vi "ExampleInstrument.TestLauncher.vi"() -> ()   [LabVIEW 2016, in "ExampleInstrument.lvclass"]
uses:
  ExampleInstrument.lvclass
  <vilib>/JKI/JKI SMO/SMO/Typedefs/SMOState --Enum.ctl
  C:/user/patrick/hg/levylab_inst/lvsrc/SMOs/Instrument/Instrument.lvclass
  C:/Program Files (x86)/National Instruments/LabVIEW 2016/vi.lib/JKI/JKI SMO/SMO/SMO.lvclass
  Example Instrument UI/ExampleInstrument.UI.lvclass
  C:/Program Files (x86)/National Instruments/LabVIEW 2016/vi.lib/JKI/JKI SMO/SMO.UI/SMO.UI.lvclass
  lvsrc/SMOs/Instrument/Instrument.lvclass/Instrument.ctl
  <vilib>/JKI/JKI SMO/SMO/SMO.lvclass
  <vilib>/JKI/JKI SMO/SMO.UI/SMO.UI.lvclass
  lvsrc/SMOs/Instrument/Instrument.lvclass
panel:
  in  "Debug Mode?":bool
  out "UI SMO State":T1
  out "SMO State":T1
  out "error out":errorcluster
  in  "Stop":bool
  # "Example Instrument SMO Test Launcher"
  # "For instructions on how to use the JKI State Machine Objects, examples and video tutorials, visit:\nhttp://jki.net/state-machine-objects/\n\nJKI State Machine Objects™\nhttp://jki.net/state-machine-objects/\nCopyright (C) 2005-2015, JKI <info@jki.net>\nALL RIGHTS RESERVED"
  # "Starting Example Instrument..."
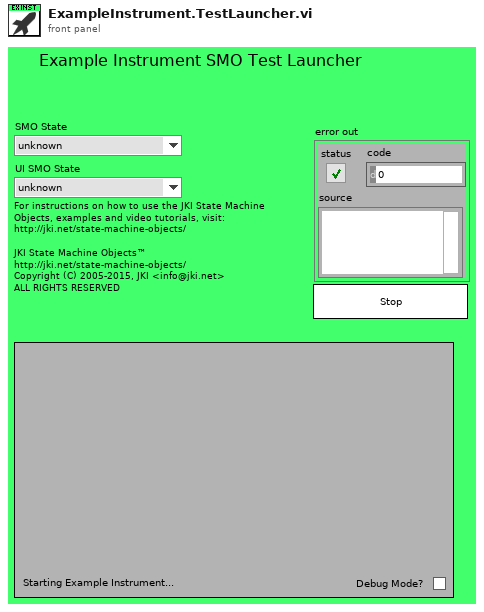
[diagram p1: front panel]
types:
  T1 = typedef "SMO.lvclass/SMOState --Enum.ctl" = enum16{"unknown", "Created", "Started", "Stopped"}
  T2 = typedef "SMO.lvclass/Public Events.ctl" = cluster{"Error":refnum<user-event>, "State":refnum<user-event>, "Reserve State":refnum<user-event>}
  T3 = cluster{"Event Registration Refnum":refnum<event-registration>, "Event Registration Refnum":refnum<event-registration>}
  T4 = enum32{"Invalid", "Standard", "Closed", "Hidden", "Minimized", "Maximized"}
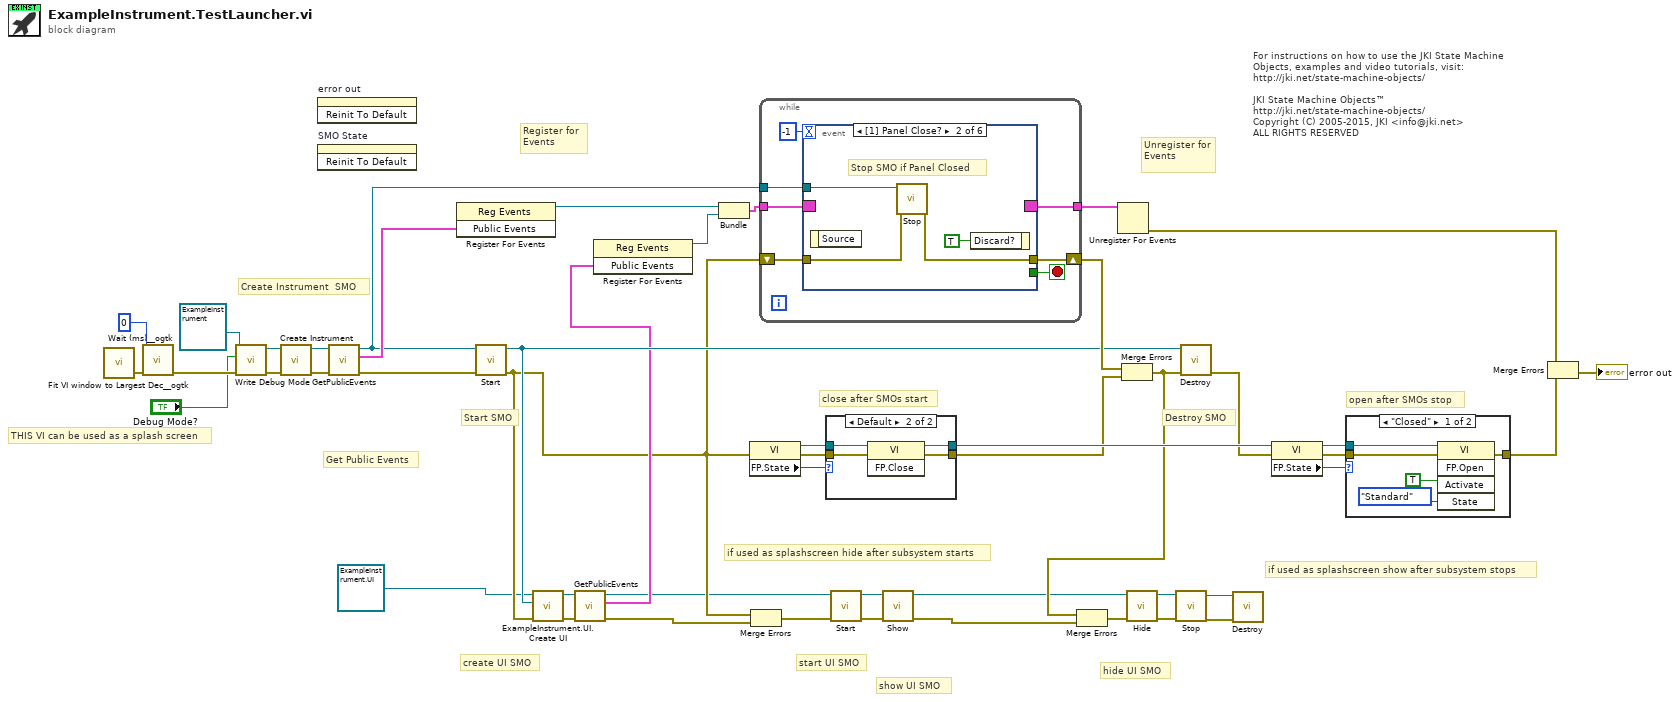
[diagram p0: block diagram]
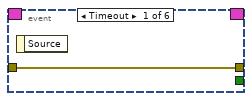
[diagram p4: hidden frame]
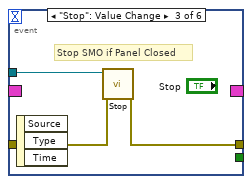
[diagram p5: hidden frame]
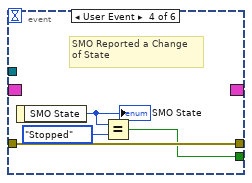
[diagram p6: hidden frame]
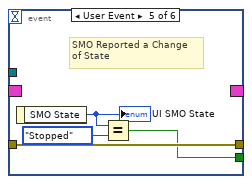
[diagram p7: hidden frame]
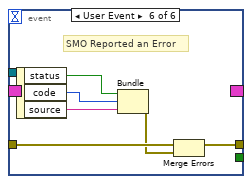
[diagram p8: hidden frame]
diagram:
  # "open after SMOs stop"
  # "close after SMOs start"
  # "hide UI SMO"
  # "show UI SMO"
  # "start UI SMO"
  # "create UI SMO"
  # "if used as splashscreen show after subsystem stops"
  # "if used as splashscreen hide after subsystem starts"
  # "THIS VI can be used as a splash screen"
  # "Get Public Events"
  # "Start SMO"
  # "Destroy SMO"
  # "Create Instrument  SMO"
  # "Unregister for Events"
  # "Register for Events"
  # "For instructions on how to use the JKI State Machine Objects, examples and video tutorials, visit:\nhttp://jki.net/state-machine-objects/\n\nJKI State Machine Objects™\nhttp://jki.net/state-machine-objects/\nCopyright (C) 2005-2015, JKI <info@jki.net>\nALL RIGHTS RESERVED"
  n1 = call <userlib>:"Fit VI window to Largest Dec__ogtk.vi"() -> ("error out"=w35:errorcluster)  [unwired: 6 in, 1 out]
  n2 = call <userlib>:"Wait (ms)__ogtk.vi"("error in (no error)"=w35, "milliseconds to wait"=u32 0) -> ("error out"=w3:errorcluster)  [unwired: 8 in, 1 out]
  n3 = call "Write Debug Mode.vi"("error in (no error)"=w3, "Debug Mode?"="Debug Mode?", "Instrument in"=refnum<class "ExampleInstrument.lvclass"> refnum ("SMO.Template.lvclass")) -> ("error out"=w2:errorcluster, "Instrument out"=w4:refnum<class "ExampleInstrument.lvclass">)  [unwired: 7 in]
  n4 = call-dynamic "Create Instrument.vi"("error in (no error)"=w2, "Instrument in"=w4) -> ("error out"=w42:errorcluster, "Instrument out"=w43:refnum<class "ExampleInstrument.lvclass">)  [unwired: 8 in]
  n5 = invoke on="error out" class="Clust (strict)" method="Reinit To Default"() -> ()  [unwired: 3 in, 3 out]
  n6 = invoke on="SMO State" class="Enum (strict)" method="Reinit To Default"() -> ()  [unwired: 3 in, 3 out]
  n7 = call <vilib>:"GetPublicEvents.vi"("error in (no error)"=w42, "SMO"=w43) -> ("error out"=w41:errorcluster, "Public Events"=w45:T2, "SMO out"=w44:refnum<class "ExampleInstrument.lvclass">)  [unwired: 7 in]
  n8 = register-events(w45) -> (reference out=w34:refnum<event-registration>)  [unwired: 2 in, 1 out]
  n9 = call <vilib>:"Start.vi"("error in (no error)"=w41, "SMO"=w44) -> ("error out"=w27:errorcluster, "SMO out"=w32:refnum<class "ExampleInstrument.lvclass">)  [unwired: 8 in]
  n10 = call "ExampleInstrument.UI.Create UI.vi"("error in (no error)"=w27, "Instrument in"=w32, "Example Instrument UI in"=refnum<class "ExampleInstrument.UI.lvclass"> refnum ("ExampleInstrument.UI.lvclass")) -> ("error out"=w30:errorcluster, "Example Instrument UI out"=w29:refnum<class "ExampleInstrument.UI.lvclass">)  [unwired: 7 in]
  n11 = call <vilib>:"GetPublicEvents.vi"("error in (no error)"=w30, "SMO"=w29) -> ("error out"=w21:errorcluster, "Public Events"=w28:T2, "SMO out"=w22:refnum<class "ExampleInstrument.UI.lvclass">)  [unwired: 7 in]
  n12 = register-events(w28) -> (reference out=w31:refnum<event-registration>)  [unwired: 2 in, 1 out]
  n13 = Bundle("Event Registration Refnum"=w34, "Event Registration Refnum"=w31) -> (w33:T3)  [unwired: 1 in]
  n14 = property class="VI"(error in=w27) -> (reference out=w12:refnum<vi>, error out=w13:errorcluster, "FP.State"=w11:T4)  [unwired: 1 in]
  n15 = Merge Errors(w27, w21) -> (w26:errorcluster)
  n16 = while {
    shift-right: [w54] -> w40
    shift-left: w27 -> [w53]
    tunnel: w33 -> [w52]
    tunnel: [w51] -> w48
    tunnel: w44 -> [w50]
    stop <- w55 stop-if-true
    n17 = event shown="[1] Panel Close?" {
      selector: w52 -> [_ _ _ _ _ _]
      dyn-events: [_ _ _ _ _ _] -> w51
      timeout: -1 -> [_ _ _ _ _ _]
      tunnel: [_ _ _ w64 w68 _] -> w55
      tunnel: w50 -> [_ w60 w63 _ _ _]
      tunnel: [w56 w59 w62 w67 w71 w75] -> w54
      tunnel: w53 -> [w56 w58 w61 w67 w71 w73]
      event Timeout {
        n18 = event-data() -> ()  [unwired: 1 in, 1 out]
      }
      event Panel Close? {
        # "Stop SMO if Panel Closed"
        n19 = event-data() -> ()  [unwired: 1 in, 1 out]
        n20 = call <vilib>:"Stop.vi"("error in (no error)"=w58, "SMO"=w60) -> ("error out"=w59:errorcluster)  [unwired: 8 in, 1 out]
        n21 = event-data("Discard?"=TRUE ("OK")) -> ()  [unwired: 1 in, 1 out]
      }
      event "Stop": Value Change {
        # "Stop SMO if Panel Closed"
        n22 = event-data() -> ()  [unwired: 1 in, 3 out]
        n23 = call <vilib>:"Stop.vi"("error in (no error)"=w61, "SMO"=w63) -> ("error out"=w62:errorcluster)  [unwired: 8 in, 1 out]
      }
      event User Event {
        # "SMO Reported a Change\nof State"
        n24 = event-data() -> ("SMO State"=w66:T1)  [unwired: 1 in]
        "SMO State" <- w66
        n25 = Equal?(x=w66, y=SMOState_--Enum."Stopped") -> (x = y?=w64:bool)
      }
      event User Event {
        # "SMO Reported a Change\nof State"
        n26 = event-data() -> ("SMO State"=w70:T1)  [unwired: 1 in]
        "UI SMO State" <- w70
        n27 = Equal?(x=w70, y=SMOState_--Enum."Stopped") -> (x = y?=w68:bool)
      }
      event User Event {
        # "SMO Reported an Error"
        n28 = event-data() -> ("status"=w74:bool, "code"=w77:i32, "source"=w76:string)  [unwired: 1 in]
        n29 = Bundle("status"=w74, "code"=w77, "source"=w76) -> (w72:errorcluster)  [unwired: 1 in]
        n30 = Merge Errors(w73, w72) -> (w75:errorcluster)
      }
    }
  }
  n31 = case shown="Default" w11 {
    tunnel: [w79 w83] -> w36
    tunnel: w13 -> [w79 w82]
    tunnel: w12 -> [w78 w81]
    tunnel: [w78 w80] -> w39
    frame "Invalid", "Closed" {
    }
    frame Default {
      n32 = invoke class="VI" method="FP.Close"(reference=w81, error in=w82) -> (reference out=w80:refnum<vi>, error out=w83:errorcluster)  [unwired: 1 in, 1 out]
    }
  }
  n33 = call <vilib>:"Start.vi"("error in (no error)"=w26, "SMO"=w22) -> ("error out"=w20:errorcluster, "SMO out"=w19:refnum<class "ExampleInstrument.UI.lvclass">)  [unwired: 8 in]
  n34 = call <vilib>:"Show.vi"("error in (no error)"=w20, "SMO.UI"=w19) -> ("error out"=w18:errorcluster, "SMO.UI out"=w14:refnum<class "ExampleInstrument.UI.lvclass">)  [unwired: 8 in]
  n35 = Unregister For Events(event registration refnum=w48) -> (error out=w47:errorcluster)  [unwired: 1 in]
  n36 = Merge Errors(w40, w36) -> (w23:errorcluster)
  n37 = Merge Errors(w23, w18) -> (w15:errorcluster)
  n38 = call <vilib>:"Hide.vi"("error in (no error)"=w15, "SMO.UI"=w14) -> ("error out"=w17:errorcluster, "SMO.UI out"=w16:refnum<class "ExampleInstrument.UI.lvclass">)  [unwired: 8 in]
  n39 = call <vilib>:"Stop.vi"("error in (no error)"=w17, "SMO"=w16) -> ("error out"=w25:errorcluster, "SMO out"=w24:refnum<class "ExampleInstrument.UI.lvclass">)  [unwired: 8 in]
  n40 = call <vilib>:"Destroy.vi"("error in (no error)"=w23, "SMO"=w32) -> ("error out"=w38:errorcluster)  [unwired: 9 in]
  n41 = call <vilib>:"Destroy.vi"("error in (no error)"=w25, "SMO"=w24) -> ()  [unwired: 9 in, 1 out]
  n42 = property class="VI"(reference=w39, error in=w38) -> (reference out=w9:refnum<vi>, error out=w10:errorcluster, "FP.State"=w8:T4)
  n43 = case shown="\"Closed\"" w8 {
    tunnel: [w86 w89] -> w37
    tunnel: w10 -> [w85 w89]
    tunnel: w9 -> [w84 _]
    frame "Closed" {
      n44 = invoke class="VI" method="FP.Open"(reference=w84, error in=w85, "Activate"=TRUE, "State"=T4."Standard") -> (error out=w86:errorcluster)  [unwired: 1 in, 4 out]
    }
    frame Default {
    }
  }
  n45 = Merge Errors(w47, w37) -> (→"error out":errorcluster)
